vi "pcap-read.vi"(0 "Opened":bool) -> (1 "Pkt Sec":i32, 2 "Pkt uSec":i32, 3 "Pkt Len":i32, 4 "Read Error":bool, 5 "Timeout":bool, 6 "Good Read":bool, 7 "Packet Data:":string)   [LabVIEW 2017]
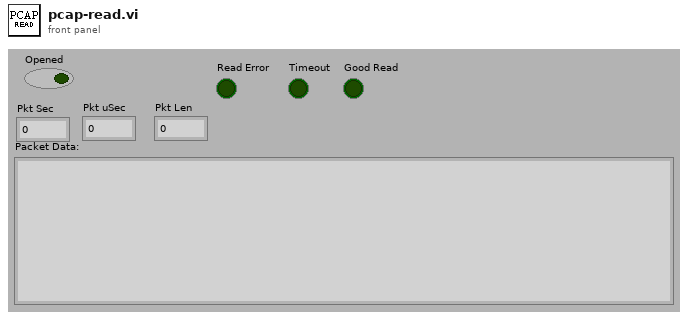
[diagram p1: front panel]
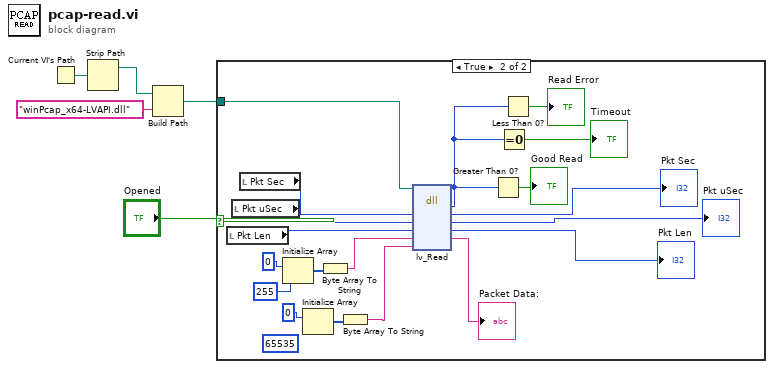
[diagram p0: block diagram]
diagram:
  n1 = Current VI's Path() -> (path=w4:path)
  n2 = Strip Path(path=w4) -> (stripped path=w3:path)  [unwired: 1 out]
  n3 = Build Path(base path=w3, name or relative path="winPcap_x64-LVAPI.dll") -> (appended path=w1:path)
  n4 = case shown="True" "Opened" {
    tunnel: w1 -> [_ w6]
    frame False {
    }
    frame True {
      (unwired) 65535
      n5 = local read "Pkt Len"() -> (w21:i32)
      n6 = local read "Pkt uSec"() -> (w22:i32)
      n7 = local read "Pkt Sec"() -> (w23:i32)
      n8 = Initialize Array(u8 0, 255) -> (w11:u8[])
      n9 = Initialize Array(u8 0) -> (w8:u8[])  [unwired: 1 in]
      n10 = Byte Array To String(unsigned byte array=w11) -> (string=w10:string)
      n11 = Byte Array To String(unsigned byte array=w8) -> (string=w7:string)
      n12 = dll-call lib="C:/Users/ucbtspu.AD/OneDrive - University College London/Local SCC/SilverLab-Microscope x64/Ethernet/winPcap_x64-LVAPI.dll" fn="lv_Read"(path in=w6, w23, w22, w21, w10, w7) -> ("return type"=w17:i32, →"Pkt Sec":i32, →"Pkt uSec":i32, →"Pkt Len":i32, →"Packet Data:":string)  [unwired: 3 in, 2 out]
      n13 = Greater Than 0?(x=w17) -> (x > 0?=→"Good Read":bool)
      n14 = Equal To 0?(x=w17) -> (x = 0?=→"Timeout":bool)
      n15 = Less Than 0?(x=w17) -> (x < 0?=→"Read Error":bool)
    }
  }
